vi "10 - Design Pattern - When Generation Rate exceeds Handling Rate (Dropped Frames).vi"() -> ()   [LabVIEW 2012]
uses:
  <vilib>/Utility/miscctls.llb/LVPoint32TypeDef.ctl
  <vilib>/Utility/miscctls.llb/LVPointTypeDef.ctl
  <vilib>/event_ctls.llb/lveventtype.ctl
panel:
  out "Canvas":picture
  out "Initial Coords":T1
  out "Events Handled per Update":dbl
  out "Events Processed":i32
  out "Most Recent Value":i32
  in  "Erase":bool
  in  "Throttler Period":u32(ring)=50 items=["50msec"=50, "500msec"=500, "None"=0]
  in  "Update Mode":T2(ring)
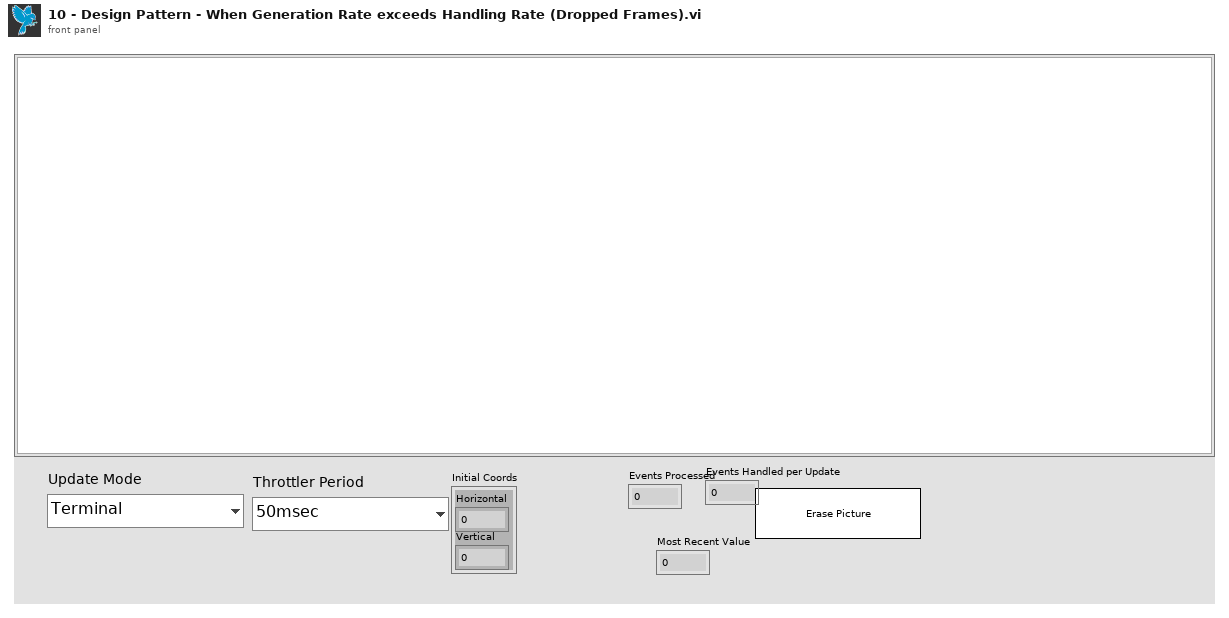
[diagram p1: front panel]
types:
  T1 = typedef "LVPoint32TypeDef.ctl" = cluster{"Horizontal":i32, "Vertical":i32}
  T2 = enum16{"Terminal", "Property Node", "Artificially Long Process"}
  T3 = typedef "LVPointTypeDef.ctl" = cluster{"Horizontal":i16, "Vertical":i16}
  T4 = enum16{"Currently Painting", "Currently Zooming", "No Action"}
  T5 = typedef "lveventtype.ctl" = enum32{"Null", "Timeout", "Annotation Menu Selection", "Annotation Menu Selection?", "App Instance Close", "App Instance Close?", "Autoscale Range Change", "Cell Edit", "Cell Edit?", "Cursor Grab", "Cursor Grab?", "Cursor Menu Selection", "Cursor Menu Selection?", "Cursor Move", "Cursor Release", "Data Change", "Direction Change", "Display State Change", "Drag Ended", "Drag Enter", "Drag Leave", "Drag Over", "Drag Source Update", "Drag Starting", "Drag Starting?", "Drop", "Exec State Change", "Key Down", "Key Down?", "Key Repeat", "Key Repeat?", "Key Up", "Listbox Double Click", "Menu Activation?", "Menu Selection (App)", "Menu Selection? (App)", "Menu Selection (User)", "Mouse Down", "Mouse Down?", "Mouse Enter", "Mouse Leave", "Mouse Move", "Mouse Up", "NI Security User Change (App)", "Pane Size", "Panel Close", "Panel Close?", "Panel Resize", "Plot Attribute Change", "Scale Range Change", "Shortcut Menu Activation?", "Shortcut Menu Selection (App)", "Shortcut Menu Selection? (App)", "Shortcut Menu Selection (User)", "Tree Double Click", "Tree Drag", "Tree Drag?", "Tree Drop", "Tree Drop?", "Tree Item Close", "Tree Item Close?", "Tree Item Open", "Tree Item Open?", "Value Change"}
  T6 = cluster{"Width":u16, "Style":enum32{"Solid", "Dash", "Dot", "DashDot", "DashDotDot"}}
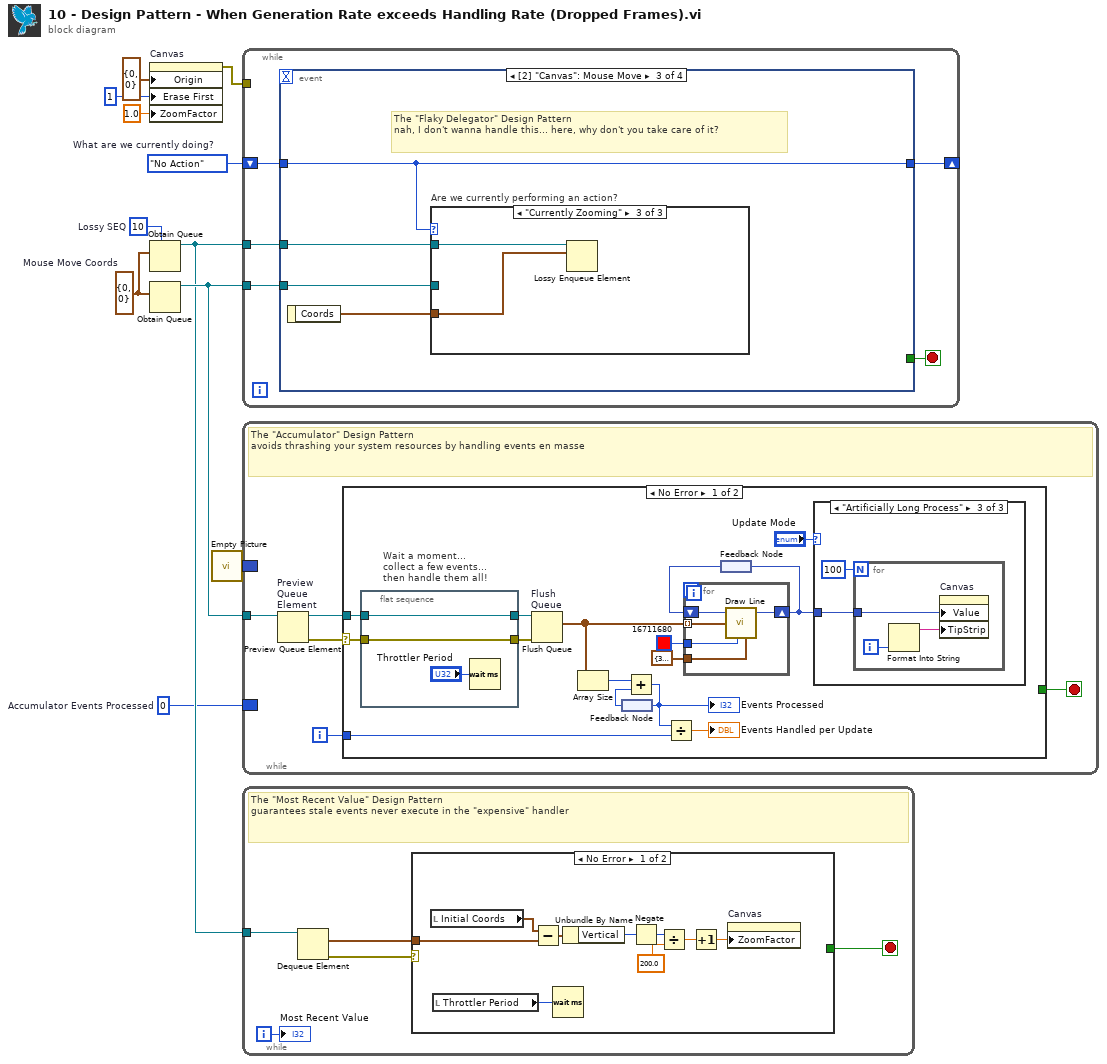
[diagram p0: block diagram]
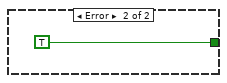
[diagram p2: hidden frame]
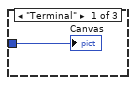
[diagram p3: hidden frame]
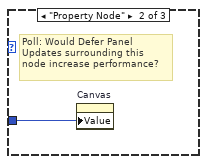
[diagram p4: hidden frame]
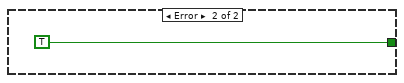
[diagram p5: hidden frame]
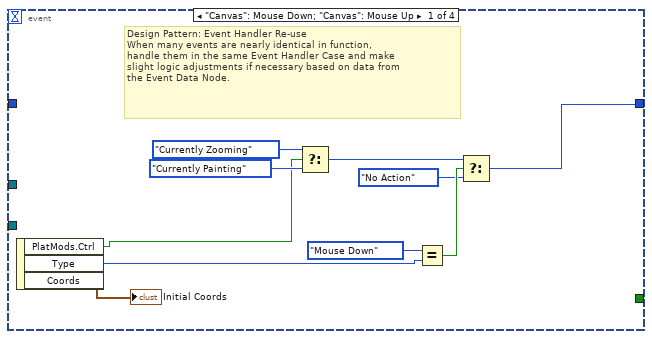
[diagram p6: hidden frame]
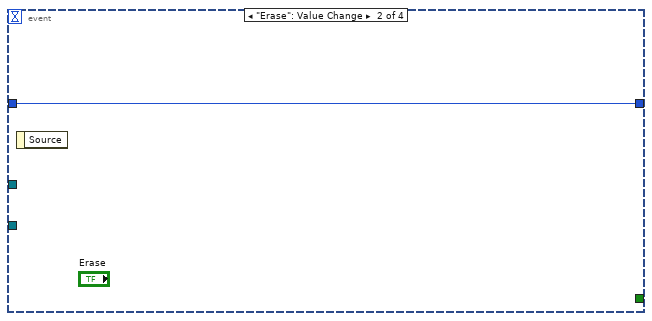
[diagram p7: hidden frame]
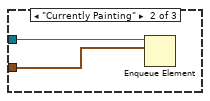
[diagram p9: hidden frame]
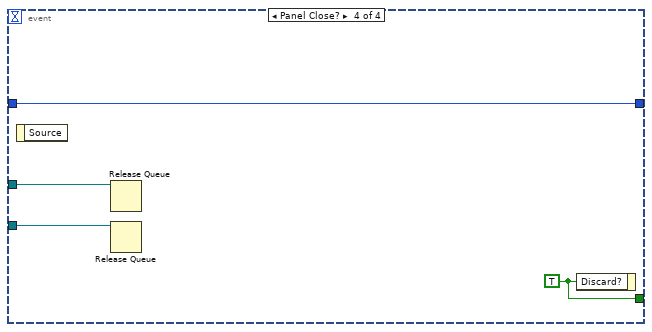
[diagram p10: hidden frame]
diagram:
  w1 = 0  # Accumulator Events Processed
  w10 = 10  # Lossy SEQ
  w11 = T4."No Action"  # What are we currently doing?
  w9 = T1 {"Horizontal"=0, "Vertical"=0}  # Mouse Move Coords
  n1 = property on="Canvas" class="Pict"("Origin"=T3 {"Horizontal"=0, "Vertical"=0}, "Erase First"=u8 1, "ZoomFactor"=sgl 1.0 ("Zoom Factor")) -> (error out=w7:errorcluster)  [unwired: 2 in, 1 out]
  n2 = Obtain Queue(max queue size (-1, unlimited)=w10, element data type=w9) -> (queue out=w4:refnum<queue>)  [unwired: 3 in, 2 out]
  n3 = Obtain Queue(element data type=w9) -> (queue out=w5:refnum<queue>)  [unwired: 4 in, 2 out]
  n4 = call "Empty Picture"() -> ("empty picture"=w6:picture)
  n5 = while {
    shift-right: [w15] -> _
    shift-left: w11 -> [w16]
    tunnel: w5 -> [w13]
    tunnel: w4 -> [w12]
    tunnel: w7 -> [_]
    stop <- w14 stop-if-true
    n6 = event shown="[2] \"Canvas\": Mouse Move" {
      selector: _ -> [_ _ _ _]
      dyn-events: _ -> [_ _ _ _]
      timeout: _ -> [_ _ _ _]
      tunnel: w16 -> [_ w27 w29 w38]
      tunnel: [w23 w27 w29 w38] -> w15
      tunnel: [_ _ _ w39] -> w14
      tunnel: w13 -> [_ _ w31 w36]
      tunnel: w12 -> [_ _ w28 w37]
      event "Canvas": Mouse Down; "Canvas": Mouse Up {
        # "Design Pattern: Event Handler Re-use\nWhen many events are nearly identical in function,\nhandle them in the same Event Handler Case and make\nslight logic adjustments if necessary based on data from\nthe Event Data Node."
        n7 = event-data() -> ("PlatMods.Ctrl"=w17:bool, "Type"=w25:T5, "Coords"=→"Initial Coords":T1)  [unwired: 1 in]
        n8 = Select(t=T4."Currently Zooming", s=w17, f=T4."Currently Painting") -> (s? t:f=w21:T4)
        n9 = Equal?(x=lveventtype."Mouse Down" ("Type"), y=w25) -> (x = y?=w24:bool)
        n10 = Select(t=w21, s=w24, f=T4."No Action") -> (s? t:f=w23:T4)
      }
      event "Erase": Value Change {
        n11 = event-data() -> ()  [unwired: 1 in, 1 out]
      }
      event "Canvas": Mouse Move {
        # "The \"Flaky Delegator\" Design Pattern\nnah, I don't wanna handle this... here, why don't you take care of it?"
        n12 = event-data() -> ("Coords"=w30:T1)  [unwired: 1 in]
        n13 = case "Are we currently performing an action?" shown="\"Currently Zooming\"" w29 {
          tunnel: w31 -> [_ w33 _]
          tunnel: w30 -> [_ w32 w35]
          tunnel: w28 -> [_ _ w34]
          frame Default {
          }
          frame "Currently Painting" {
            n14 = Enqueue Element(queue=w33, element=w32) -> ()  [unwired: 2 in, 3 out]
          }
          frame "Currently Zooming" {
            n15 = Lossy Enqueue Element(queue=w34, element=w35) -> ()  [unwired: 1 in, 4 out]
          }
        }
      }
      event Panel Close? {
        w39 = TRUE ("Discard?")
        n16 = event-data() -> ()  [unwired: 1 in, 1 out]
        n17 = Release Queue(queue=w37) -> ()  [unwired: 2 in, 3 out]
        n18 = Release Queue(queue=w36) -> ()  [unwired: 2 in, 3 out]
        n19 = event-data("Discard?"=w39) -> ()  [unwired: 1 in, 1 out]
      }
    }
  }
  n20 = while {
    tunnel: w5 -> [w44]
    border: w6 -> [_]
    border: w1 -> [_]
    i -> [w40]
    stop <- w41 stop-if-true
    # "The \"Accumulator\" Design Pattern\navoids thrashing your system resources by handling events en masse"
    n21 = Preview Queue Element "Preview\nQueue\nElement"(queue=w44) -> (queue out=w42:refnum<queue>, error out=w43:errorcluster)  [unwired: 2 in, 2 out]
    n22 = case shown="No Error" w43 {
      selector: w43 -> [w58 _]
      tunnel: w42 -> [w57 _]
      tunnel: [_ TRUE] -> w41
      tunnel: w40 -> [w46 _]
      frame No Error {
        n23 = flat-sequence "Wait a moment...\ncollect a few events...\nthen handle them all!" {
          tunnel: [w74] -> w59
          tunnel: w58 -> [w74]
          tunnel: w57 -> [w73]
          tunnel: [w73] -> w56
          frame #0 {
            n24 = Wait (ms)(milliseconds to wait="Throttler Period") -> ()  [unwired: 1 out]
          }
        }
        n25 = Flush Queue "Flush\nQueue"(queue=w56, error in (no error)=w59) -> (remaining elements=w52:T1[])  [unwired: 2 out]
        n26 = Array Size(array=w52) -> (size(s)=w51:i32)
        n27 = feedback #1() -> (w50:i32)
        n28 = Add(x=w51, y=w50) -> (x+y=w47:i32)
        "Events Processed" <- w47
        n29 = feedback-in #1(w47) -> ()
        n30 = Divide(x=w47, y=w46) -> (x/y=→"Events Handled per Update":dbl)
        n31 = feedback #2() -> (w53:picture)
        n32 = for {
          shift-right: [w71] -> w54
          shift-left: w53 -> [w70]
          tunnel: w52 -> [w69] mode=indexing
          tunnel: u32 16711680 ("color(black)") -> [w68]
          tunnel: T6 {"Width"=3, "Style"=enum."Solid"} ("pen") -> [w67]
          n33 = call <vilib>:"Draw Line.vi"("picture"=w70, "end point"=w69, "color(black)"=w68, "pen"=w67) -> ("new picture"=w71:picture)  [unwired: 5 in]
        }
        n34 = feedback-in #2(w54) -> ()
        n35 = case shown="\"Artificially Long Process\"" "Update Mode" {
          tunnel: w54 -> [w60 w61 w63]
          frame "Terminal" {
            "Canvas" <- w60
          }
          frame "Property Node" {
            # "Poll: Would Defer Panel\nUpdates surrounding this\nnode increase performance?"
            n36 = property on="Canvas" class="Pict"("Value"=w61) -> ()  [unwired: 2 in, 2 out]
          }
          frame "Artificially Long Process" {
            n37 = for {
              N: 100 ("Numeric") -> [_]
              tunnel: w63 -> [w66]
              i -> [w65]
              n38 = Format Into String(w65) -> (resulting string=w64:string)  [unwired: 3 in, 1 out]
              n39 = property on="Canvas" class="Pict"("Value"=w66, "TipStrip"=w64) -> ()  [unwired: 2 in, 2 out]
            }
          }
        }
      }
      frame Error {
      }
    }
  }
  n40 = while {
    tunnel: w4 -> [w80]
    i -> [w76]
    stop <- w77 stop-if-true
    # "The \"Most Recent Value\" Design Pattern\nguarantees stale events never execute in the \"expensive\" handler"
    n41 = Dequeue Element(queue=w80) -> (element=w78:T1, error out=w79:errorcluster)  [unwired: 2 in, 2 out]
    n42 = case shown="No Error" w79 {
      tunnel: w78 -> [w89 _]
      tunnel: [_ TRUE] -> w77
      frame No Error {
        n43 = local read "Initial Coords"() -> (w82:T1)
        n44 = local read "Throttler Period"() -> (w86:u32)
        n45 = Subtract(x=w82, y=w89) -> (x-y=w88:T1)
        n46 = Wait (ms)(milliseconds to wait=w86) -> ()  [unwired: 1 out]
        n47 = Unbundle By Name(w88) -> ("Vertical"=w83:i32)
        n48 = Negate(x=w83) -> (-x=w81:i32)
        n49 = Divide(x=w81, y=200.0) -> (x/y=w87:dbl)
        n50 = Increment(x=w87) -> (x+1=w84:dbl)
        n51 = property on="Canvas" class="Pict"("ZoomFactor"=w84) -> ()  [unwired: 2 in, 2 out]
      }
      frame Error {
      }
    }
    "Most Recent Value" <- w76
  }
